vi "fake THz module.vi"(10 "Main controller mailbox":T4, 11 "THz module mailbox":T4) -> ()   [LabVIEW 2022 SP3, in "THz source modeule.lvlib"]
uses:
  THz source modeule.lvlib
  Messenger service/Data types/Mailbox address.ctl
  ctl/THz MW generator constants.ctl
  ctl/VDI status.ctl
  ctl/Synth status.ctl
  Messenger service/Data types/Module name.ctl
  ctl/THz sweep parameters.ctl
  ctl/THz Message for module.ctl
  ctl/THz commands enum.ctl
  <vilib>/ErrorRing/Error Ring.xnode
  Messenger service/MessengerLib.lvlib
panel:
  in  "Status in":T1={"Master"={"Mode"=enum."CW", "Conected"=TRUE}, "Follower"={"Mode"=enum."CW", "Conected"=TRUE}}
  out "Ended":bool
  out "?":T3[](array[typedef])=[{"Lower limit [GHz]"=8.0, "Upper limit [GHz]"=20.0, "Device name"="VDIS0122", "Connection"="123", "Description"="VDI Synth", "Connected"=TRUE, "Last settings"="", "Operation mode"=enum."Disabled", "Enable ch 1"=FALSE, "Enable ch 2"=FALSE}, {"Lower limit [GHz]"=8.0, "Upper limit [GHz]"=20.0, "Device name"="VDIYT7", "Connection"="321", "Description"="VDI Tracking", "Connected"=TRUE, "Last settings"="", "Operation mode"=enum."Disabled", "Enable ch 1"=FALSE, "Enable ch 2"=FALSE}]
  out "Initialized":bool
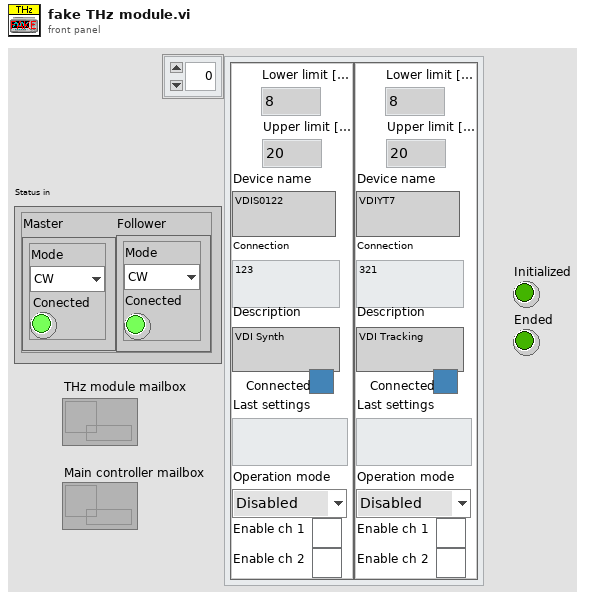
[diagram p1: front panel]
types:
  T1 = typedef "THz source modeule.lvlib/VDI status.ctl" = cluster{"Master":T2, "Follower":T2}
  T2 = typedef "THz source modeule.lvlib/Synth status.ctl" = cluster{"Mode":enum16{"CW", "Sweep"}, "Conected":bool}
  T3 = typedef "THz source modeule.lvlib/THz MW generator constants.ctl" = cluster{"Lower limit [GHz]":dbl, "Upper limit [GHz]":dbl, "Device name":string, "Connection":string, "Description":string, "Connected":bool, "Last settings":string, "Operation mode":enum16{"Disabled", "CW", "Arbitrary", "Sweep"}, "Enable ch 1":bool, "Enable ch 2":bool}
  T4 = typedef "MessengerLib.lvlib/Mailbox address.ctl" = refnum<queue>
  T5 = typedef "Module name.ctl" = enum16{"Emty", "Magnet", "VTI", "Excitation", "Servo", "Acquisition", "Rotator", "Digitizer", "SMU2450", "Carousel", "Multimeter", "Tmp monitor", "Power monitor"}
  T6 = typedef "THz source modeule.lvlib/THz sweep parameters.ctl" = cluster{"Start [GHz]":dbl, "End [GHz] ":dbl, "Sweep up\ntime [ms]":dbl, "Sweep down\ntime [ms]":dbl, "Intermidiate [MHz]":dbl, "Reset trigger":bool}
  T7 = typedef "THz source modeule.lvlib/THz commands enum.ctl" = enum16{"Ignore", "Connect", "Update", "Set parameters", "Disconnect", "End"}
  T8 = typedef "THz source modeule.lvlib/THz Message for module.ctl" = cluster{"Command":T7, "Data":variant}
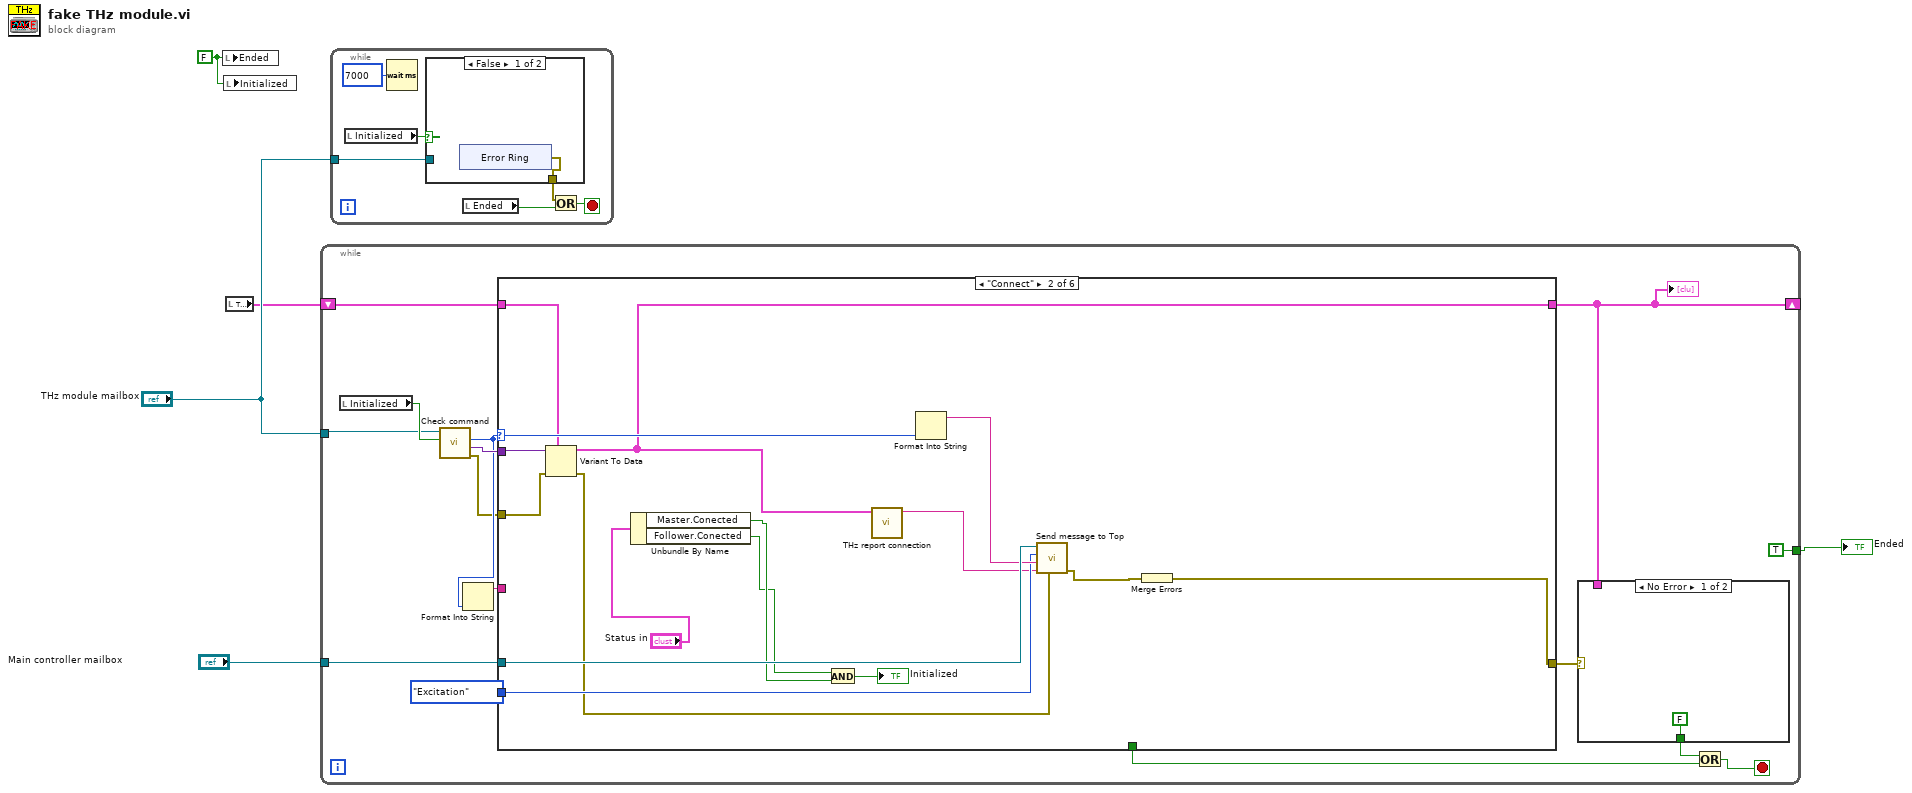
[diagram p0: block diagram]
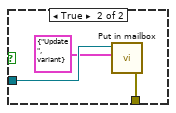
[diagram p2: hidden frame]
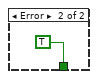
[diagram p3: hidden frame]
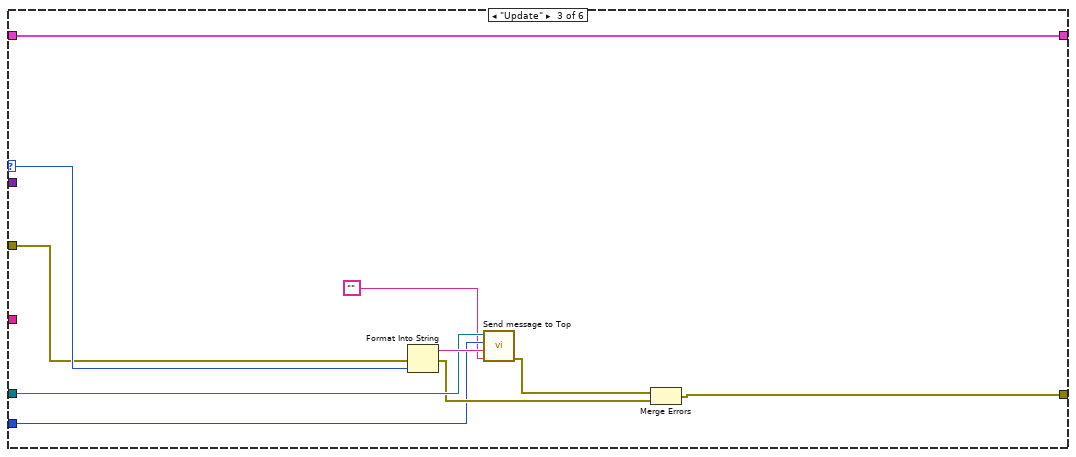
[diagram p5: hidden frame]
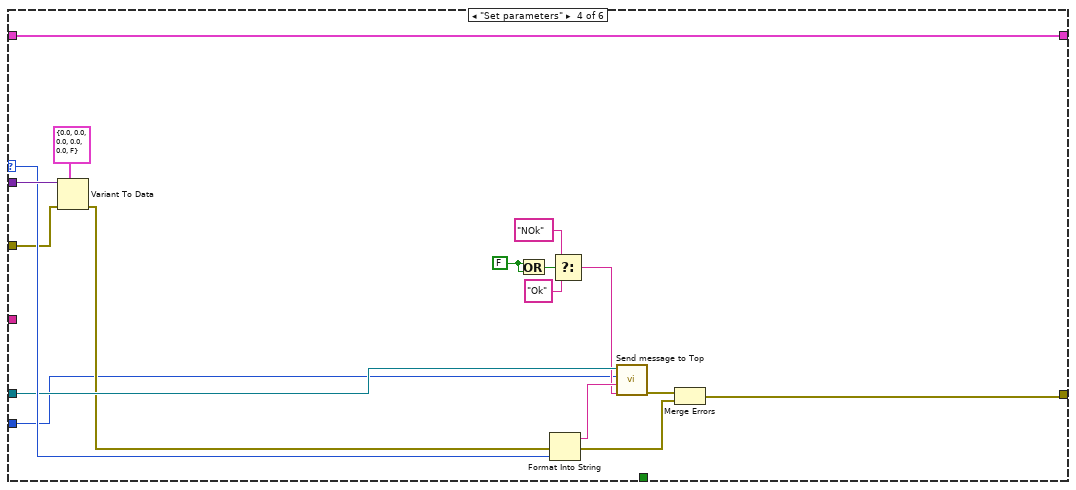
[diagram p6: hidden frame]
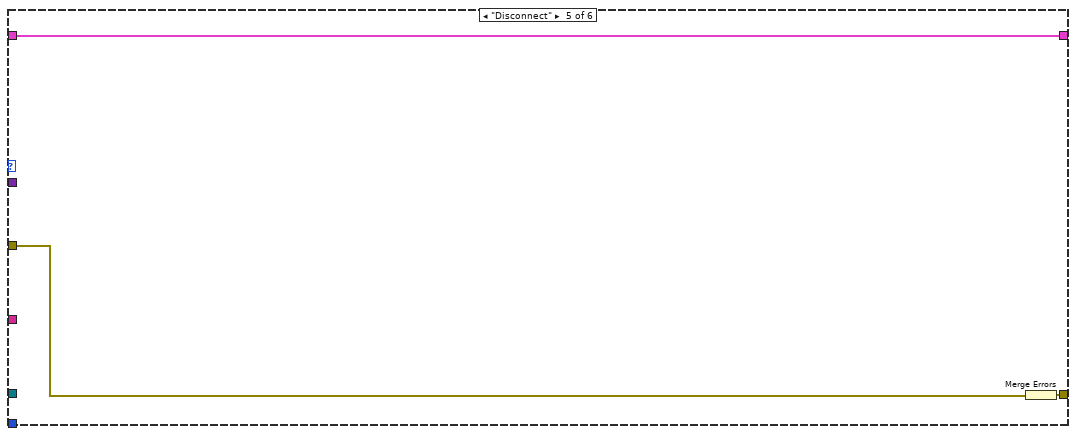
[diagram p7: hidden frame]
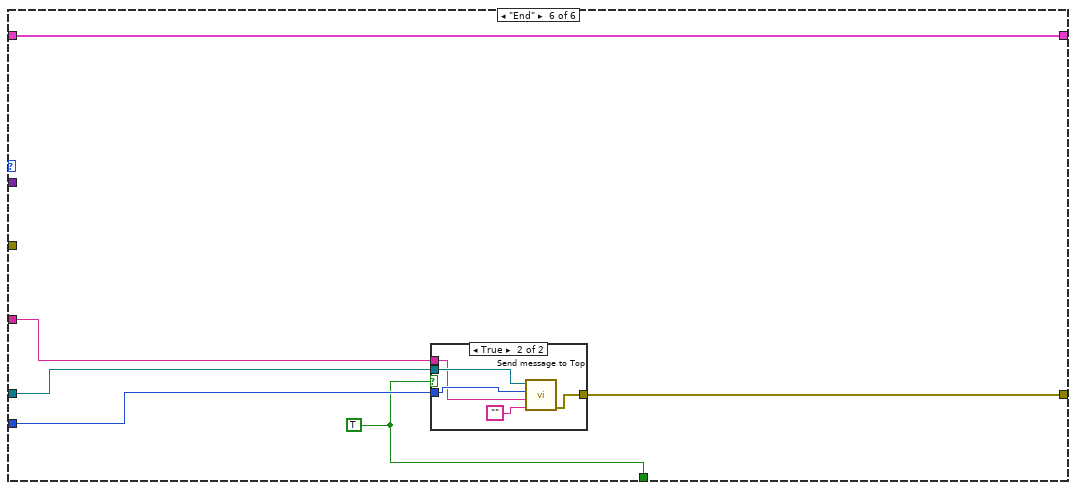
[diagram p8: hidden frame]
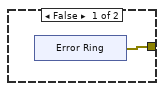
[diagram p9: hidden frame]
diagram:
  w1 = FALSE ("Initialized")
  n1 = local write "Ended"(w1) -> ()
  n2 = local write "Initialized"(w1) -> ()
  n3 = local read item#3() -> (w3:T3[])
  n4 = while {
    shift-right: [w16] -> _
    shift-left: w3 -> [w20]
    tunnel: "THz module mailbox" -> [w7]
    tunnel: "Main controller mailbox" -> [w19]
    tunnel: [TRUE ("Initialized")] -> w2
    stop <- w14 stop-if-true
    n5 = local read "Initialized"() -> (w17:bool)
    n6 = call "Check command.vi"("Is connected"=w17, "Module mailbox"=w7) -> ("error out"=w6:errorcluster, "Command Data"=w18:variant, "Command"=w9:T7)  [unwired: 3 in]
    n7 = Format Into String(w9) -> (resulting string=w8:string)  [unwired: 3 in, 1 out]
    n8 = case shown="\"Connect\"" w9 {
      selector: w9 -> [_ w39 w49 w63 _ _]
      tunnel: [w24 w28 w43 w66 w70 w72] -> w16
      tunnel: w20 -> [w24 w32 w43 w66 w70 w72]
      tunnel: w18 -> [_ w40 _ w67 _ _]
      tunnel: [_ _ _ _ _ w71] -> w15
      tunnel: w19 -> [_ w38 w48 w62 _ w76]
      tunnel: [w23 w35 w46 w55 w68 w75] -> w11
      tunnel: w6 -> [w23 w33 w45 w57 w69 _]
      tunnel: Module_name."Excitation" ("Module") -> [_ w31 w42 w52 _ w74]
      tunnel: w8 -> [_ _ _ _ _ w73]
      frame "Ignore", Default {
      }
      frame "Connect" {
        n9 = Variant To Data(error in=w33, type=w32, Variant=w40) -> (data=w28:T3[], error out=w29:errorcluster)
        n10 = Unbundle By Name("Status in") -> ("Master.Conected"=w27:bool, "Follower.Conected"=w26:bool)
        n11 = And(x=w26, y=w27) -> (x .and. y?=→"Initialized":bool)
        n12 = call "THz report connection.vi"("THz MW generator constants"=w28) -> ("string out"=w25:string)  [unwired: 10 in]
        n13 = Format Into String(w39) -> (resulting string=w37:string)  [unwired: 3 in, 1 out]
        n14 = call "Send message to Top.vi"("Error in (no error)"=w29, "Data"=w25, "Response"=w37, "Module"=w31, "Mailbox address in"=w38) -> ("Error out"=w34:errorcluster)  [unwired: 5 in, 1 out]
        n15 = Merge Errors(w34) -> (w35:errorcluster)
      }
      frame "Update" {
        n16 = Format Into String(error in=w45, w49) -> (resulting string=w50:string, error out=w44:errorcluster)  [unwired: 2 in]
        n17 = call "Send message to Top.vi"("Data"="", "Response"=w50, "Module"=w42, "Mailbox address in"=w48) -> ("Error out"=w47:errorcluster)  [unwired: 6 in, 1 out]
        n18 = Merge Errors(w47, w44) -> (w46:errorcluster)
      }
      frame "Set parameters" {
        w51 = FALSE ("x")
        n19 = Variant To Data(error in=w57, type=T6 {"Start [GHz]"=0.0, "End [GHz] "=0.0, "Sweep up\ntime [ms]"=0.0, "Sweep down\ntime [ms]"=0.0, "Intermidiate [MHz]"=0.0, "Reset trigger"=FALSE} ("Sweep parameters"), Variant=w67) -> (error out=w56:errorcluster)  [unwired: 1 out]
        n20 = Or(x=w51, y=w51) -> (x .or. y?=w61:bool)
        n21 = Format Into String(error in=w56, w63) -> (resulting string=w64:string, error out=w54:errorcluster)  [unwired: 2 in]
        n22 = Select(t="NOk", s=w61, f="Ok") -> (s? t:f=w59:string)
        n23 = call "Send message to Top.vi"("Data"=w59, "Response"=w64, "Module"=w52, "Mailbox address in"=w62) -> ("Error out"=w53:errorcluster)  [unwired: 6 in, 1 out]
        n24 = Merge Errors(w53, w54) -> (w55:errorcluster)
      }
      frame "Disconnect" {
        n25 = Merge Errors(w69) -> (w68:errorcluster)
      }
      frame "End" {
        w71 = TRUE
        n26 = case shown="True" w71 {
          tunnel: w76 -> [_ w83]
          tunnel: [w77 w82] -> w75
          tunnel: w74 -> [_ w80]
          tunnel: w73 -> [_ w79]
          frame False {
            n27 = xnode "Error Ring"() -> ("error out"=w77:errorcluster)
          }
          frame True {
            n28 = call "Send message to Top.vi"("Data"="", "Response"=w79, "Module"=w80, "Mailbox address in"=w83) -> ("Error out"=w82:errorcluster)  [unwired: 6 in, 1 out]
          }
        }
      }
    }
    "?" <- w16
    n29 = case shown="No Error" w11 {
      tunnel: w16 -> [_ _]
      tunnel: [FALSE TRUE] -> w13
      frame No Error {
      }
      frame Error {
      }
    }
    n30 = Or(x=w13, y=w15) -> (x .or. y?=w14:bool)
  }
  "Ended" <- w2
  n31 = while {
    tunnel: "THz module mailbox" -> [w87]
    stop <- w86 stop-if-true
    n32 = local read "Initialized"() -> (w88:bool)
    n33 = Wait (ms)(milliseconds to wait=u32 7000) -> ()  [unwired: 1 out]
    n34 = case shown="False" w88 {
      tunnel: w87 -> [_ w94]
      tunnel: [w90 w92] -> w85
      frame False {
        n35 = xnode "Error Ring"() -> ("error out"=w90:errorcluster)
      }
      frame True {
        n36 = call "Put in mailbox.vi"("Message"=T8 {"Command"=enum."Update", "Data"=variant} ("Incoming msg"), "Queue in"=w94) -> ("error out"=w92:errorcluster)  [unwired: 7 in, 2 out]
      }
    }
    n37 = local read "Ended"() -> (w84:bool)
    n38 = Or(x=w85, y=w84) -> (x .or. y?=w86:bool)
  }
